vi "semester_1_project_global.vi"() -> ()   [LabVIEW 2024]
panel:
  in  "Sample Rate Control":dbl
  in  "Humidity setpoint low control":dbl
  in  "Humidity setpoint high control":dbl
  in  "Temperature setpoint low control":dbl
  in  "Power Switch":bool
  in  "Temperature setpoint high control":dbl
  out "Historical Humidity":dbl[](graph)
  out "Historical Temperature":dbl[](graph)
  out "Humidity Running Avg":dbl
  out "Temperature Running Avg":dbl
  out "Humidity 6":dbl
  out "Humidity 5":dbl
  out "Humidity 4":dbl
  out "Humidity 3":dbl
  out "Humidity 2":dbl
  out "Humidity 1":dbl
  out "Temperature 6":dbl
  out "Temperature 5":dbl
  out "Temperature 4":dbl
  out "Temperature 3":dbl
  out "Temperature 2":dbl
  out "Temperature 1":dbl
  out "Humidity Min":dbl
  out "Humidity Max":dbl
  out "Temperature Min":dbl
  out "Temperature Max":dbl
  out "Humidity setpoint high":dbl
  out "Humidity setpoint low":dbl
  out "Temperature setpoint high":dbl
  out "Temperature setpoint low":dbl
  out "Dehumidifier":bool
  out "Heater":bool
  out "Power":bool
  out "Sample Rate":dbl
  out "Humidity":dbl(slide) scale=0.0..100.0
  out "Temperature":dbl(slide) scale=0.0..100.0
  # "Indicators"
  # "Controls"
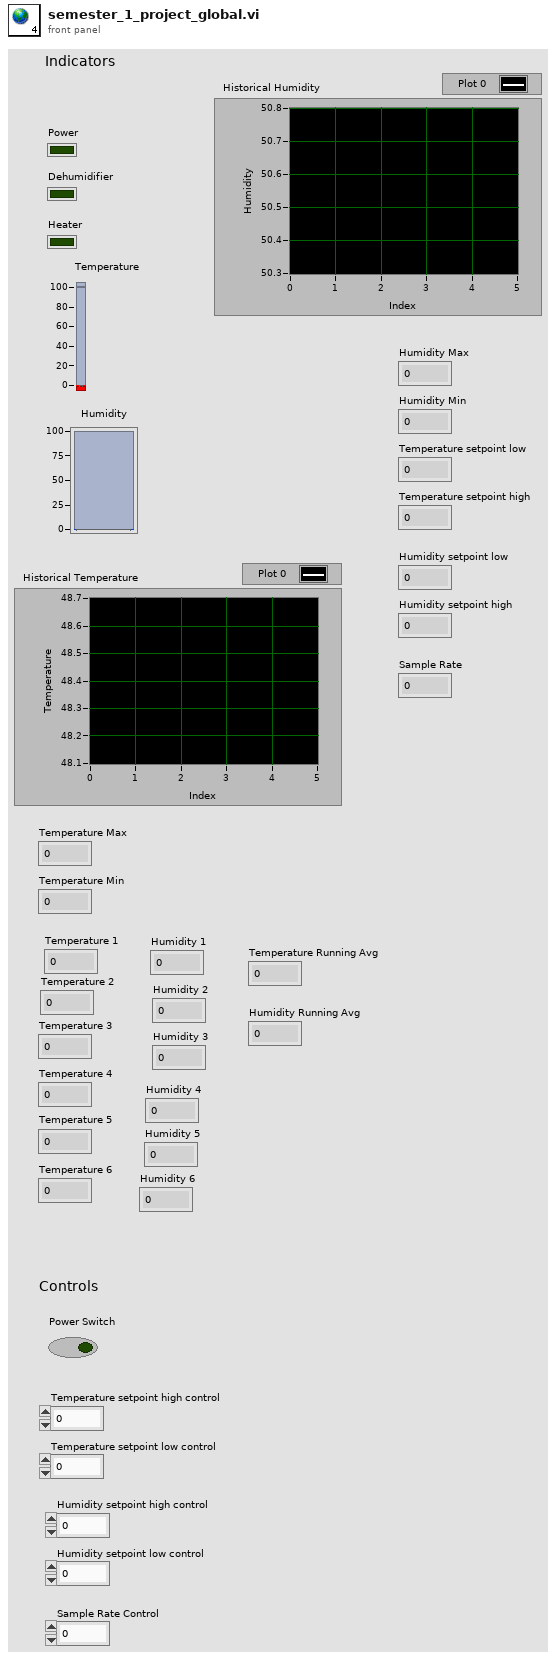
[diagram p1: front panel]
diagram:
